vi "Sub Initialize.vi"(8 "error in (no error)":errorcluster, 11 "Spectrum Recorder in":refnum<class "Spectrum Recorder too.lvclass">) -> (0 "error out":errorcluster, 2 "Initialize Result":refnum<class "Acquired Result.lvclass">, 3 "Spectrum Recorder out":refnum<class "Spectrum Recorder too.lvclass">)   [LabVIEW 2016, in "Spectrum Recorder too.lvclass"]
uses:
  Spectrum Recorder too.lvclass
  C:/github/Measure_core/Worker/Worker.lvclass
  C:/github/Measure_core/Instrument Actor/Instrument Actor.lvclass
  Measure_core/Results/Acquired Result/Acquired Result.lvclass
  Measure_core/Worker/Worker.lvclass/Worker.ctl
  Spectrum Recorder too.lvclass/Spectrum Recorder too.ctl
  Measure_core/Template Module/Write Active.vi
  Measure_core/Template Module/Read Active.vi
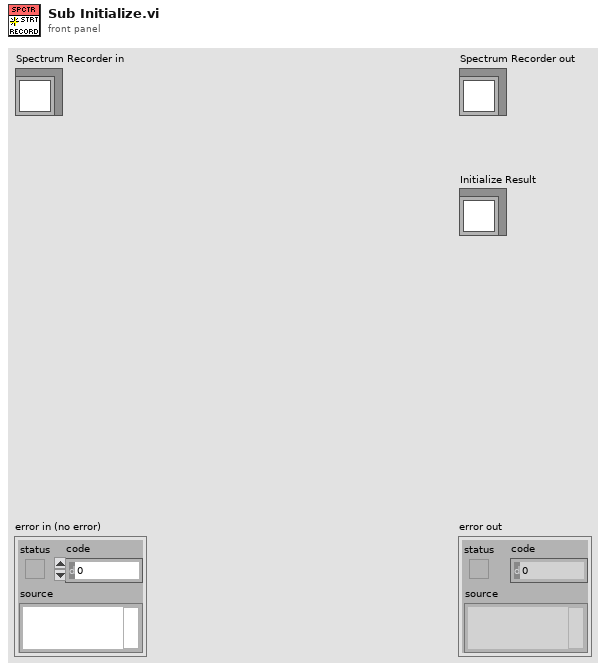
[diagram p1: front panel]
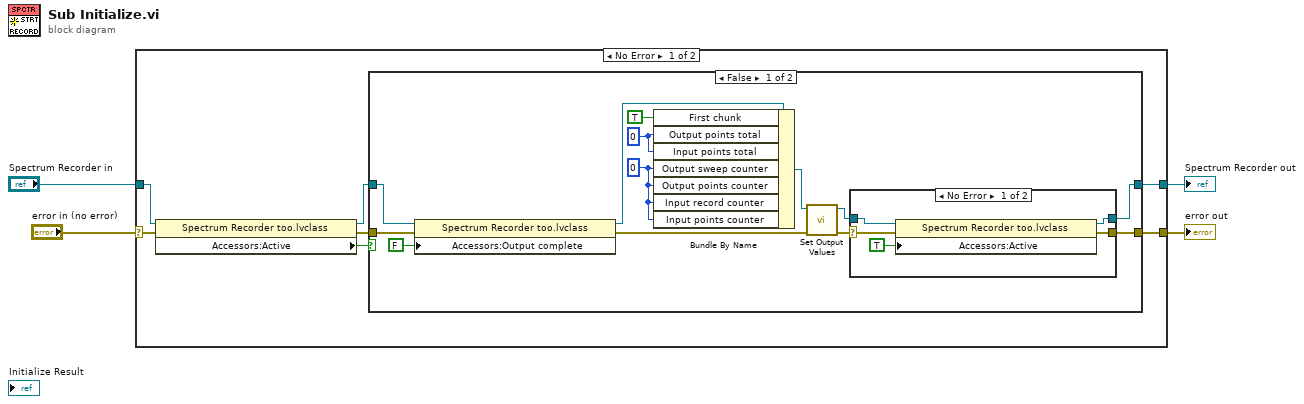
[diagram p0: block diagram]
diagram:
  n1 = case shown="No Error" "error in (no error)" {
    selector: "error in (no error)" -> [w6 w35]
    tunnel: [w9 w35] -> w3
    tunnel: [w11 w34] -> w1
    tunnel: "Spectrum Recorder in" -> [w10 w34]
    frame No Error {
      n2 = property class="Spectrum Recorder too.lvclass"(reference=w10, error in=w6) -> (reference out=w8:refnum<class "Spectrum Recorder too.lvclass">, error out=w5:errorcluster, "Accessors:Active"=w7:bool)
      n3 = case shown="False" w7 {
        tunnel: w8 -> [w16 w33]
        tunnel: [w18 w33] -> w11
        tunnel: w5 -> [w14 w32]
        tunnel: [w23 w32] -> w9
        frame False {
          w17 = i64 0 ("Output points total")
          w22 = 0 ("Output sweep counter")
          n4 = property class="Spectrum Recorder too.lvclass"(reference=w16, error in=w14, "Accessors:Output complete"=FALSE ("Output complete")) -> (reference out=w15:refnum<class "Spectrum Recorder too.lvclass">, error out=w13:errorcluster)
          n5 = Bundle By Name(cluster=w15, "First chunk"=TRUE, "Output points total"=w17, "Input points total"=w17, "Output sweep counter"=w22, "Output points counter"=w22, "Input record counter"=w22, "Input points counter"=w22) -> (w24:refnum<class "Spectrum Recorder too.lvclass">)
          n6 = call-dynamic "Set Output Values.vi"("error in (no error)"=w13, "Spectrum Recorder in"=w24) -> ("error out"=w20:errorcluster, "Spectrum Recorder out"=w19:refnum<class "Spectrum Recorder too.lvclass">)  [unwired: 8 in]
          n7 = case shown="No Error" w20 {
            selector: w20 -> [w29 w30]
            tunnel: [w25 w30] -> w23
            tunnel: w19 -> [w28 w31]
            tunnel: [w27 w31] -> w18
            frame No Error {
              n8 = property class="Spectrum Recorder too.lvclass"(reference=w28, error in=w29, "Accessors:Active"=TRUE ("Value")) -> (reference out=w27:refnum<class "Spectrum Recorder too.lvclass">, error out=w25:errorcluster)
            }
            frame Error {
            }
          }
        }
        frame True {
        }
      }
    }
    frame Error {
    }
  }
  "error out" <- w3
  "Spectrum Recorder out" <- w1
